vi "Test Prepare Path Returns Default File Name if Folder Given.vi"(11 "Test Case In":refnum<class "Report Plugin Test.lvclass">) -> (0 "error out":errorcluster, 3 "Test Case Out":refnum<class "Report Plugin Test.lvclass">)   [LabVIEW 2020, in "Report Plugin Test.lvclass"]
uses:
  Report Plugin Test.lvclass
  C:/git/astemes-lunit/source/Framework/Report Plugin/Report Plugin.lvclass
  C:/Program Files (x86)/National Instruments/LabVIEW 2020/vi.lib/Astemes/LUnit/Test Case.lvclass
  <vilib>/Astemes/LUnit/Test Case.lvclass/Test Case.ctl
  e1eeebb6-1c69-40ac-a018-3a09ac31808e.vi
  <vilib>/Astemes/LUnit/Core/LUnit Test Case/Private/Append Pass Result.vi
  <vilib>/Astemes/LUnit/Core/LUnit Test Case/Private/Append Fail Result.vi
  e1eeebb6-1c69-40ac-a018-3a09ac31808e.vi/9c5d11cd-9439-4240-a1ee-d9baace9c924.vi
  <vilib>/Astemes/LUnit/Core/LUnit Test Case/Private/Run In UI.vi
  <vilib>/Utility/error.llb/Clear Errors.vi
  source/Framework/Report Plugin/Report Plugin.lvclass
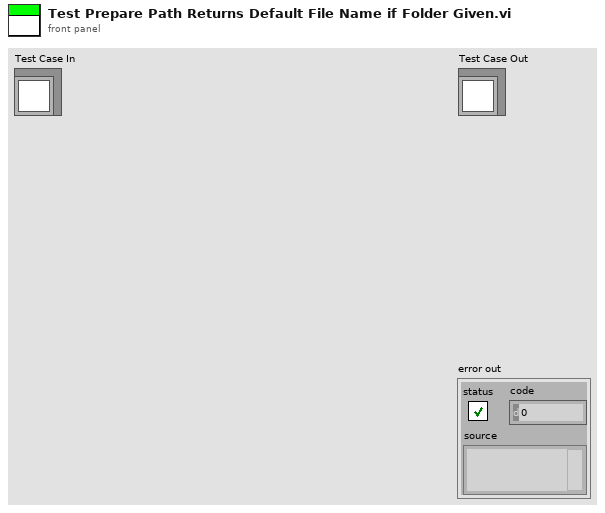
[diagram p1: front panel]
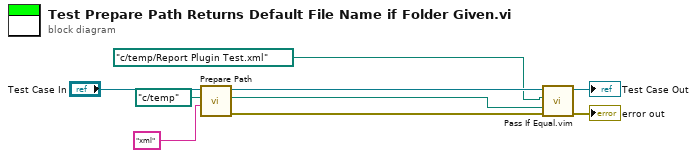
[diagram p0: block diagram]
diagram:
  n1 = call "Prepare Path.vi"("Extenssion"="xml", "File Path in"=path "c:/temp", "Plugin In"="Test Case In") -> ("error out"=w5:errorcluster, "Modified Path"=w4:path, "Plugin Out"=w6:refnum<class "Report Plugin Test.lvclass">)  [unwired: 6 in]
  n2 = call "Pass If Equal.vim"("error in (no error)"=w5, "Actual"=w4, "Expected"=path "c:/temp/Report Plugin Test.xml" ("File Path in"), "LUnit Test Case In"=w6) -> ("error out"=→"error out":errorcluster, "LUnit Test Case Out"=→"Test Case Out":refnum<class "Report Plugin Test.lvclass">)  [unwired: 6 in]
